vi "stringFilter.vi"(8 "error in":errorcluster, 9 "Active":bool, 10 "filterString":string, 11 "inputString":string) -> (0 "error out":errorcluster, 3 "resultString":string)   [LabVIEW 2018]
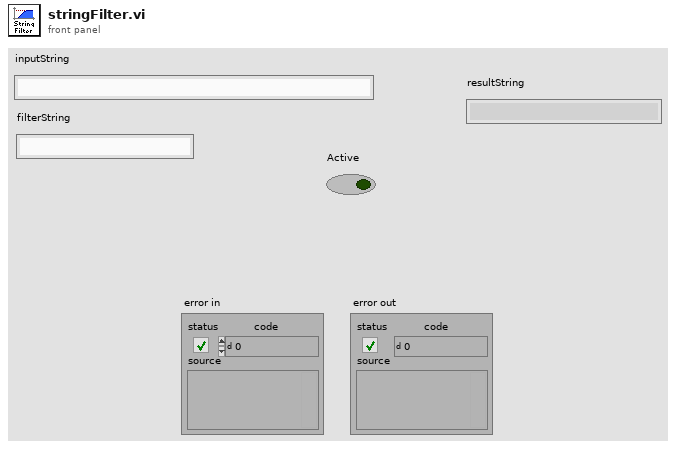
[diagram p1: front panel]
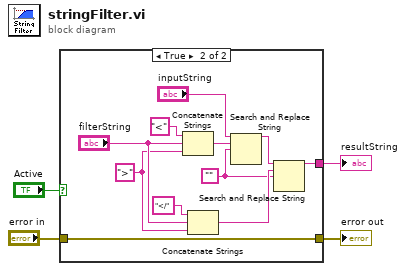
[diagram p0: block diagram]
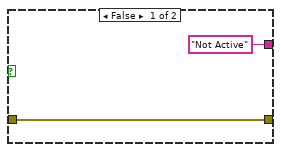
[diagram p2: hidden frame]
diagram:
  n1 = case shown="True" "Active" {
    tunnel: "error in" -> [w6 w8]
    tunnel: [w6 w8] -> w2
    tunnel: ["Not Active" ("result string") w7] -> w1
    frame False {
    }
    frame True {
      w9 = ""
      w11 = ">" ("string")
      n2 = Concatenate Strings("<" ("string"), "filterString", w11) -> (w14:string)
      n3 = Concatenate Strings("</" ("string"), "filterString", w11) -> (w16:string)
      n4 = Search and Replace String(input string="inputString", search string=w14, replace string=w9) -> (result string=w15:string)  [unwired: 5 in, 3 out]
      n5 = Search and Replace String(input string=w15, search string=w16, replace string=w9) -> (result string=w7:string)  [unwired: 5 in, 3 out]
    }
  }
  "error out" <- w2
  "resultString" <- w1
